vi "Write Analogue.vi"(8 "error in (no error)":errorcluster, 9 "output":bool, 10 "Channel index(0)":i32, 11 "NI Fgen in":refnum<class "NI Fgen.lvclass">) -> (0 "error out":errorcluster, 2 "Success?":bool, 3 "NI Fgen out":refnum<class "NI Fgen.lvclass">)   [LabVIEW 2025, in "Fgen.lvlib" / "NI Fgen.lvclass"]
uses:
  NI Fgen.lvclass
  NI Fgen.lvclass/NI Fgen.ctl
  400085ca-fd83-4753-8dfc-9719c7c2b8a3.vi
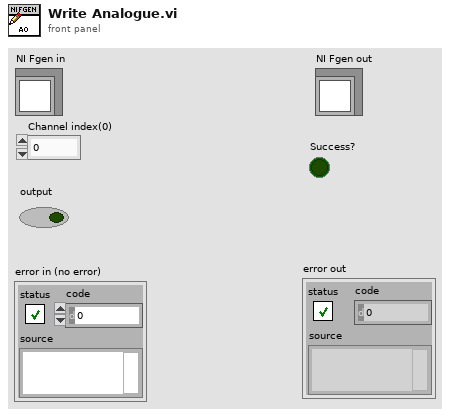
[diagram p1: front panel]
types:
  T1 = typedef "Abstract Engine.lvlibp/Abstract Instrument.lvclass/Channel.ctl" = cluster{"Index":i32, "Alias":string, "Unit":T2, "Upper limit":dbl, "Lower limit":dbl, "Measurement":variant}
  T2 = typedef "Abstract Engine.lvlibp/Abstract Instrument.lvclass/Unit.ctl" = enum16{"V", "A", "Ohm", "Hz", "uF", "degC", "deg"}
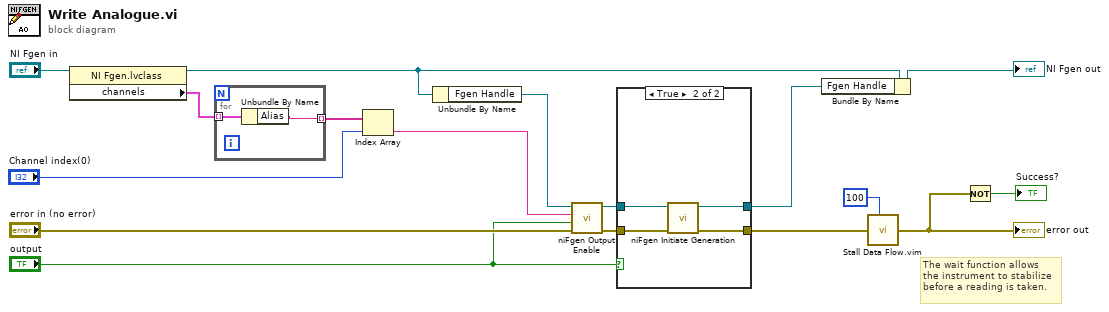
[diagram p0: block diagram]
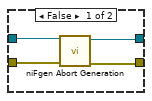
[diagram p2: hidden frame]
diagram:
  # "The wait function allows \nthe instrument to stabilize\nbefore a reading is taken."
  n1 = property class="NI Fgen.lvclass"(reference="NI Fgen in") -> (reference out=w3:refnum<class "NI Fgen.lvclass">, "channels"=w2:T1[])  [unwired: 1 in, 1 out]
  n2 = for {
    tunnel: w2 -> [w19] mode=indexing
    tunnel: [w18] -> w1 mode=indexing
    n3 = Unbundle By Name(w19) -> ("Alias"=w18:string)
  }
  n4 = Index Array(array=w1, index="Channel index(0)") -> (element=w4:string)
  n5 = Unbundle By Name(w3) -> ("Fgen Handle"=w12:refnum<k15>)
  n6 = call <instrlib>:"niFgen Output Enable.vi"("error in (no error)"="error in (no error)", "Output Enable (default: True)"="output", "Channel Name"=w4, "Instrument Handle"=w12) -> ("error out"=w14:errorcluster, "Instrument Handle Out"=w15:refnum<k15>)  [unwired: 6 in]
  n7 = case shown="True" "output" {
    tunnel: w14 -> [w23 w27]
    tunnel: w15 -> [w21 w26]
    tunnel: [w22 w25] -> w17
    tunnel: [w20 w24] -> w8
    frame False {
      n8 = call <instrlib>:"niFgen Abort Generation.vi"("error in (no error)"=w23, "Instrument Handle"=w21) -> ("error out"=w22:errorcluster, "Instrument Handle Out"=w20:refnum<k15>)  [unwired: 8 in]
    }
    frame True {
      n9 = call <instrlib>:"niFgen Initiate Generation.vi"("error in (no error)"=w27, "Instrument Handle"=w26) -> ("error out"=w25:errorcluster, "Instrument Handle Out"=w24:refnum<k15>)  [unwired: 8 in]
    }
  }
  n10 = Bundle By Name(cluster=w3, "Fgen Handle"=w8) -> (→"NI Fgen out":refnum<class "NI Fgen.lvclass">)
  n11 = call "Stall Data Flow.vim"("value in"=w17, "milliseconds to wait"=u32 100 ("millisecond timer value")) -> ("value out"=w7:errorcluster)  [unwired: 1 out]
  "error out" <- w7
  n12 = Not(x=w7) -> (.not. x?=→"Success?":bool)
